vi "Refactor Dependencies for VI.vi"(8 "error in":errorcluster, 10 "rename data":T3, 11 "vi reference in":refnum<vi>) -> (0 "error out":errorcluster, 1 "missing dependencies":bool, 2 "missing items":T2, 3 "vi reference out":refnum<vi>)   [LabVIEW 2021, in "MeasurementService Editor.lvlib"]
uses:
  MeasurementService Editor.lvlib
  Rename Refactor Data.ctl
  Rename Refactor Mapping Info.ctl
  Rename String Mapping.ctl
  Refactor Object Result.ctl
  <vilib>/Utility/traverseref.llb/TRef TravTarget.ctl
  <vilib>/Utility/traverseref.llb/VI Scripting - Traverse.lvlib
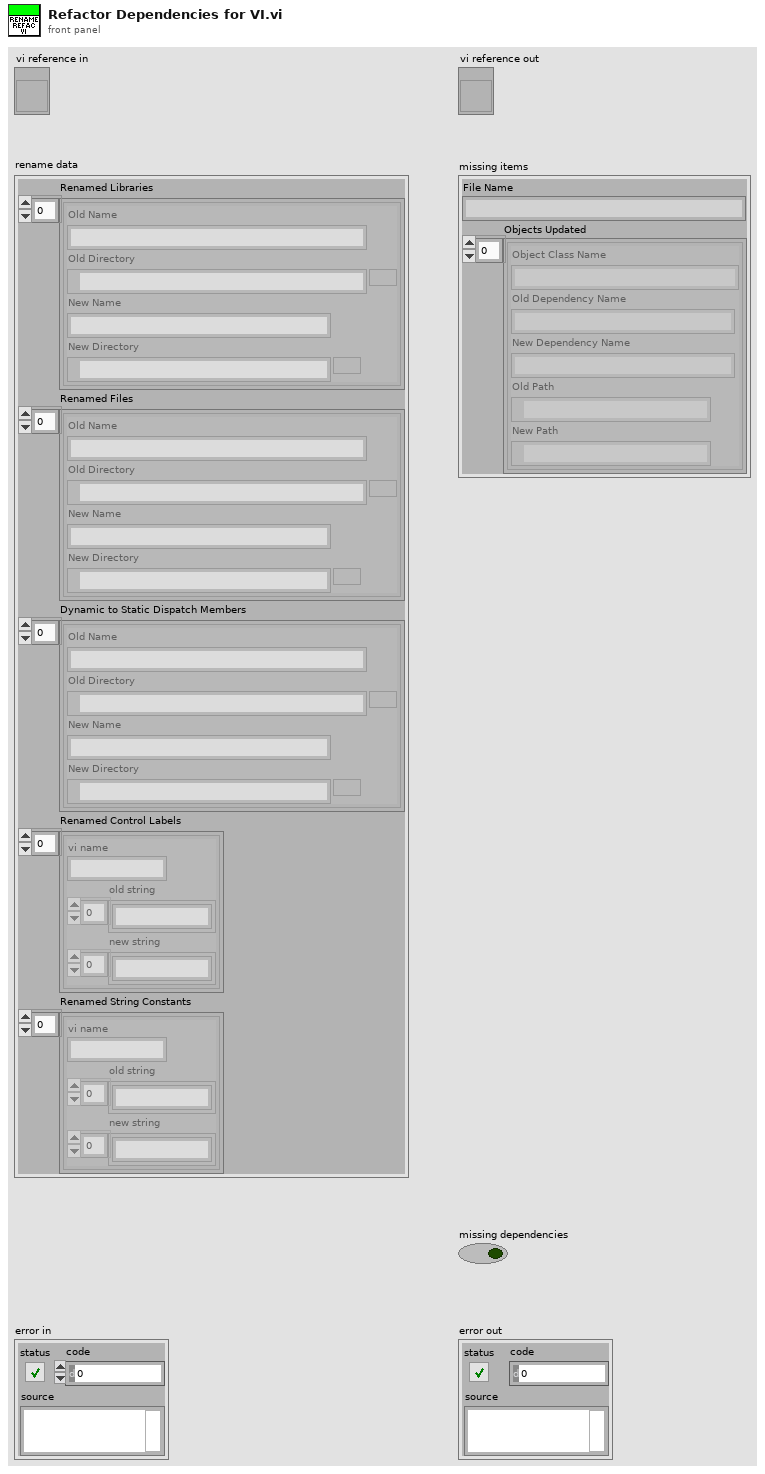
[diagram p1: front panel]
types:
  T1 = typedef "MeasurementService Editor.lvlib/Refactor Object Result.ctl" = cluster{"Object Class Name":string, "Old Dependency Name":string, "New Dependency Name":string, "Old Path":path, "New Path":path}
  T2 = cluster{"File Name":string, "Objects Updated":T1[]}
  T3 = typedef "MeasurementService Editor.lvlib/Rename Refactor Data.ctl" = cluster{"Renamed Libraries":T4[], "Renamed Files":T4[], "Dynamic to Static Dispatch Members":T4[], "Renamed Control Labels":T5[], "Renamed String Constants":T5[]}
  T4 = typedef "MeasurementService Editor.lvlib/Rename Refactor Mapping Info.ctl" = cluster{"Old Name":string, "Old Directory":path, "New Name":string, "New Directory":path}
  T5 = typedef "MeasurementService Editor.lvlib/Rename String Mapping.ctl" = cluster{"vi name":string, "old string":string[], "new string":string[]}
  T6 = typedef "TRef TravTarget.ctl" = enum16{"FP", "BD", "Other"}
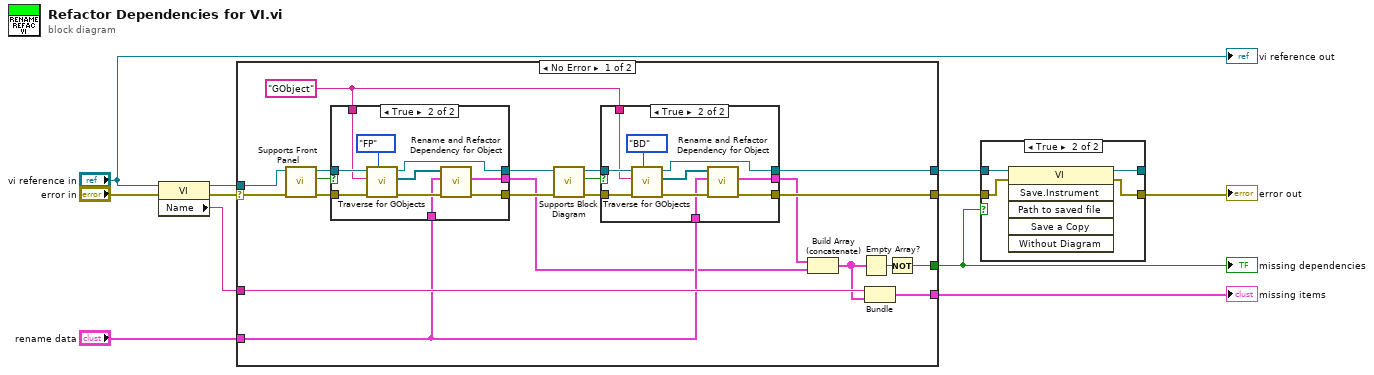
[diagram p0: block diagram]
diagram:
  n1 = property class="VI"(reference="vi reference in", error in="error in") -> (reference out=w10:refnum<vi>, error out=w9:errorcluster, "Name"=w11:string)
  n2 = case shown="No Error" w9 {
    selector: w9 -> [w28 w58]
    tunnel: [w32 _] -> w6
    tunnel: [w31 _] -> w7
    tunnel: w11 -> [w30 _]
    tunnel: w10 -> [w29 w57]
    tunnel: [w27 w58] -> w5
    tunnel: [w26 w57] -> w4
    tunnel: "rename data" -> [w14 _]
    frame No Error {
      w24 = "GObject" ("Class Name")
      n3 = call "Supports Front Panel.vi"("error in (no error)"=w28, "vi in"=w29) -> ("error out"=w20:errorcluster, "has front panel"=w21:bool, "vi out"=w22:refnum<vi>)  [unwired: 7 in]
      n4 = case shown="True" w21 {
        tunnel: w22 -> [w46 w54]
        tunnel: [w46 w47] -> w18
        tunnel: [w45 w53] -> w19
        tunnel: w24 -> [_ w52]
        tunnel: [_ w51] -> w12
        tunnel: w20 -> [w45 w50]
        tunnel: w14 -> [_ w48]
        frame False {
          # "poly VIs don't have front panels"
        }
        frame True {
          n5 = call <vilib>:"Traverse for GObjects.vi"("Traverse Target"=TRef_TravTarget."FP", "error in (no error)"=w50, "Class Name"=w52, "VI Refnum"=w54) -> ("error out"=w56:errorcluster, "References"=w49:refnum<vi>[], "dup VI Refnum"=w47:refnum<vi>)  [unwired: 4 in, 1 out]
          n6 = call "Rename and Refactor Dependency for Object.vi"("error in (no error)"=w56, "rename data"=w48, "object references"=w49) -> ("error out"=w53:errorcluster, "refactor results"=w51:T1[])  [unwired: 7 in]
        }
      }
      n7 = call "Supports Block Diagram.vi"("error in (no error)"=w19, "vi in"=w18) -> ("error out"=w15:errorcluster, "has block diagram"=w16:bool, "vi out"=w17:refnum<vi>)  [unwired: 7 in]
      n8 = case shown="True" w16 {
        tunnel: w17 -> [w33 w43]
        tunnel: w24 -> [_ w42]
        tunnel: [w34 w37] -> w27
        tunnel: [w33 w36] -> w26
        tunnel: w15 -> [w34 w41]
        tunnel: w14 -> [_ w38]
        tunnel: [_ w35] -> w13
        frame False {
        }
        frame True {
          n9 = call <vilib>:"Traverse for GObjects.vi"("Traverse Target"=TRef_TravTarget."BD", "error in (no error)"=w41, "Class Name"=w42, "VI Refnum"=w43) -> ("error out"=w40:errorcluster, "References"=w39:refnum<vi>[], "dup VI Refnum"=w36:refnum<vi>)  [unwired: 4 in, 1 out]
          n10 = call "Rename and Refactor Dependency for Object.vi"("error in (no error)"=w40, "rename data"=w38, "object references"=w39) -> ("error out"=w37:errorcluster, "refactor results"=w35:T1[])  [unwired: 7 in]
        }
      }
      n11 = Build Array (concatenate)(w13, w12) -> (w23:T1[])
      n12 = Empty Array?(array=w23) -> (empty?=w25:bool)
      n13 = Bundle("Name"=w30, w23) -> (w31:cluster{"Name":string, T1[]})  [unwired: 1 in]
      n14 = Not(x=w25) -> (.not. x?=w32:bool)
    }
    frame Error {
    }
  }
  "missing dependencies" <- w6
  "missing items" <- w7
  n15 = case shown="True" w6 {
    tunnel: w5 -> [w60 w63]
    tunnel: [w60 w61] -> w1
    tunnel: w4 -> [w59 w64]
    tunnel: [w59 w62] -> _
    frame False {
    }
    frame True {
      n16 = invoke class="VI" method="Save.Instrument"(reference=w64, error in=w63) -> (reference out=w62:refnum<vi>, error out=w61:errorcluster)  [unwired: 4 in, 4 out]
    }
  }
  "error out" <- w1
  "vi reference out" <- "vi reference in"
